vi "TCP Server - Parse message.vi"(6 "Sender IP":string, 8 "error in (no error)":errorcluster, 9 "Message":string, 10 "TCP Client ID":refnum<k5>, 11 "TCP Server in":refnum<class "TCP Server.lvclass">) -> (0 "error out":errorcluster, 1 "External error out":errorcluster, 3 "TCP Server out":refnum<class "TCP Server.lvclass">)   [LabVIEW 2026, in "TALOS.lvlib" / "TCP Server.lvlib" / "TCP Server.lvclass"]
uses:
  TCP Server.lvclass
  TCP Server Msg Actions.ctl
  Ancestor/Ancestor/Ancestor.lvclass/Ancestor.ctl
  <vilib>/Utility/error.llb/Trim Whitespace (string).vi
  <vilib>/Utility/error.llb/Trim Whitespace One-Sided.vi
  FGV/Error Memory/Get Error Description.vi
  Ancestor/Ancestor/Read ID.vi
  Support VIs/Get Class Name.vi
  <vilib>/Utility/error.llb/Clear Errors.vi
  FGV/Error Memory/Error Memory Core.vi
  <vilib>/AdvancedString/Delimited String to 1D String Array.vi
  <vilib>/AdvancedString/Delimited String to 1D String Array (string).vi
  Support VIs/Circus Root Path.vi
  FGV/Error Memory/Error Crt Lvl checker.vi
  FGV/Error Memory/Error Memory Core.vi/40c8088d-b597-4017-91af-faa98e00292e.vi
  FGV/Error Memory/Error Memory Core.vi/d4a3ab98-063c-4e44-b43d-fbdcfe6c2be2.vi
  Support VIs/Global Constants.vi
  Support VIs/Global Memory.vi
  <userlib>/_OpenG.lib/string/string.llb/Trim Whitespace (String)__ogtk.vi
  <vilib>/Utility/LVClass/Get LV Class Name.vi
  Support VIs/Is in Packed Library.vi
  Support VIs/TALOS Root path.vi
  Support VIs/Read CSV worksheet.vi
  <vilib>/Utility/error.llb/General Error Handler.vi
  Support VIs/Error Log.vi
  Ancestor/Ancestor/Ancestor.lvclass
  <vilib>/Comparison/Equal/Equal Functor/Equal Functor.lvclass
  bd90c6b7-bc86-460d-9dd7-41153e43b143.vi
  TALOS.lvlib
  <userlib>/_OpenG.lib/string/string.llb/openg_string.lvlib
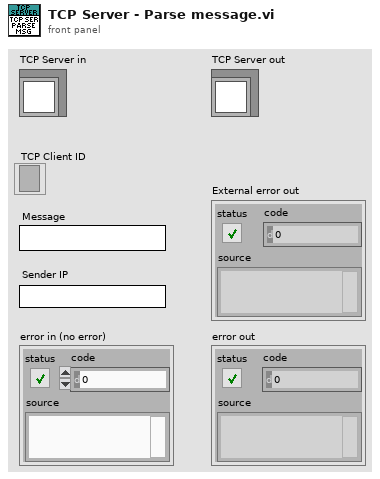
[diagram p1: front panel]
types:
  T1 = typedef "TALOS.lvlib/TCP Server.lvlib/TCP Server.lvclass/TCP Server Msg Actions.ctl" = enum16{"Spawn TCP Listener/Writer", "External Error", "I Exist", "Who the hell is this guy?", "Do nothing", "Are you the Bearer", "Farewell", "External Message"}
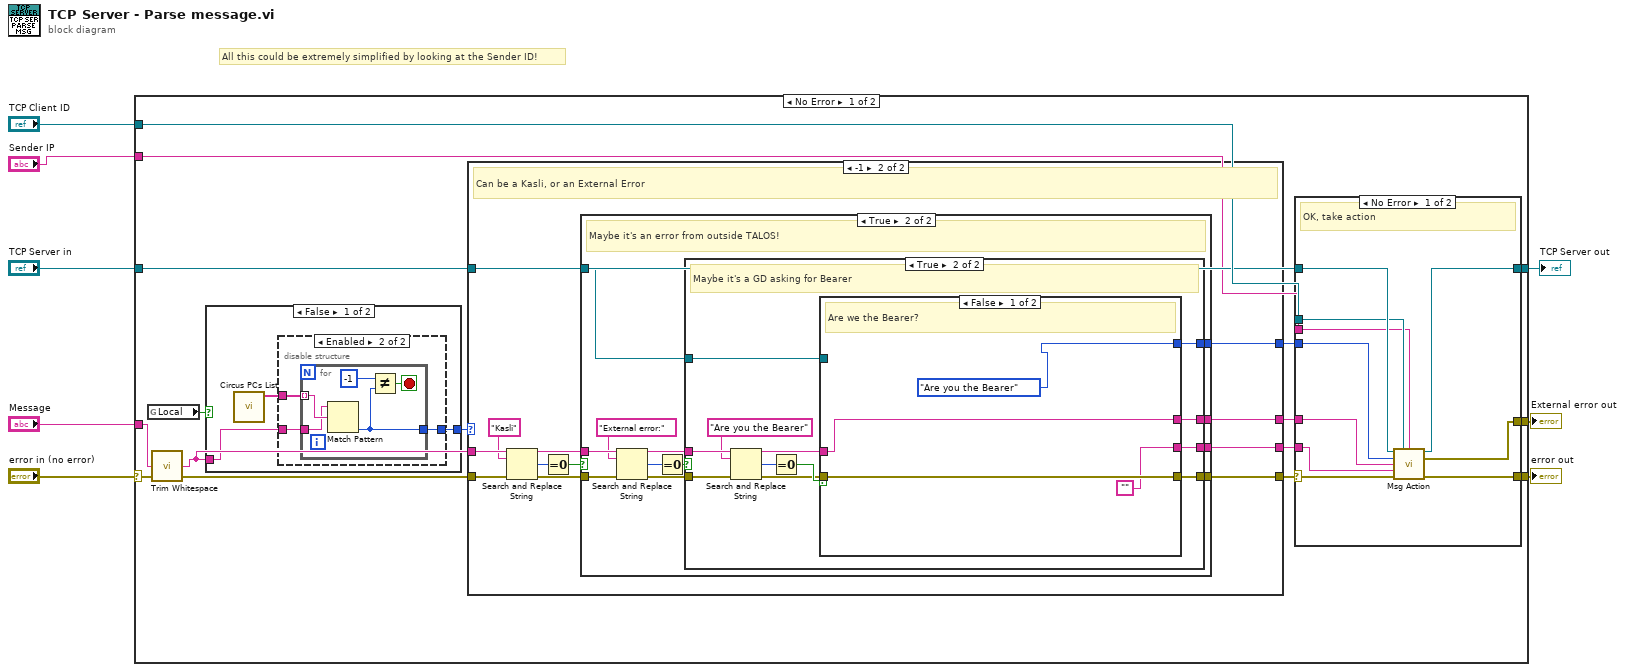
[diagram p0: block diagram]
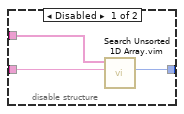
[diagram p2: hidden frame]
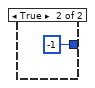
[diagram p3: hidden frame]
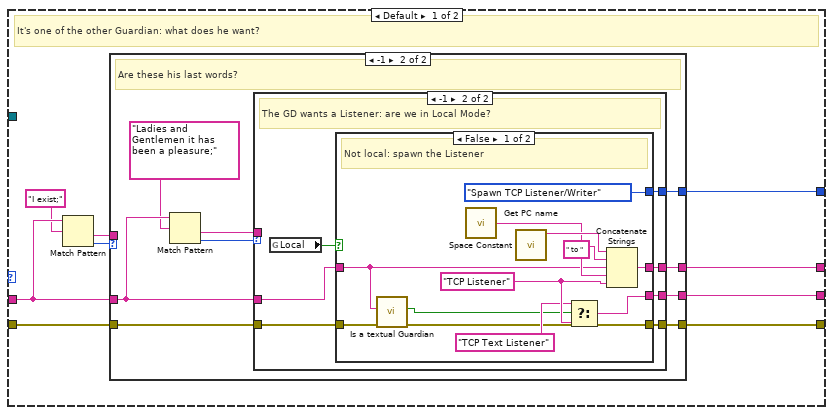
[diagram p4: hidden frame]
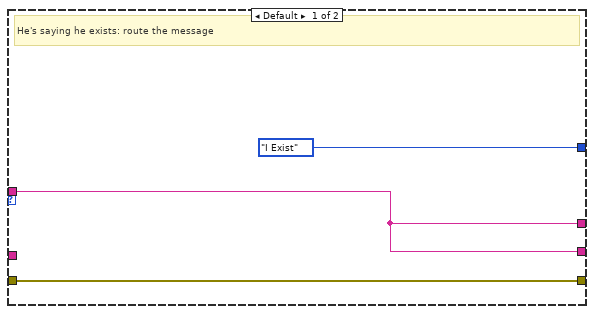
[diagram p5: hidden frame]
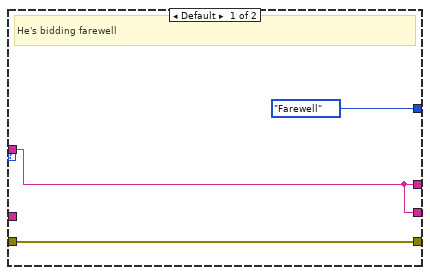
[diagram p6: hidden frame]
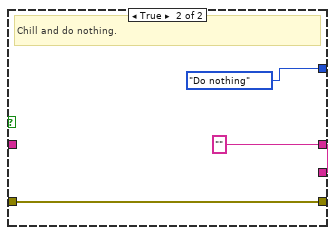
[diagram p7: hidden frame]
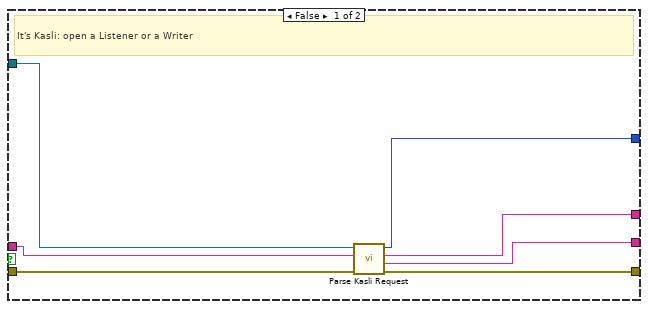
[diagram p8: hidden frame]
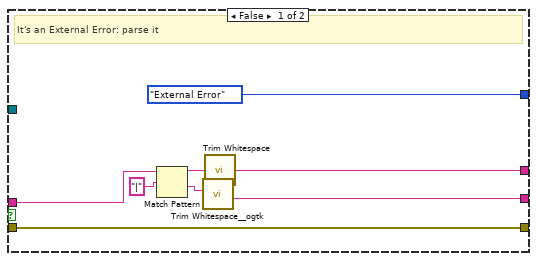
[diagram p9: hidden frame]
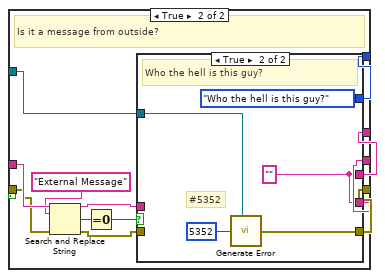
[diagram p10: hidden frame]
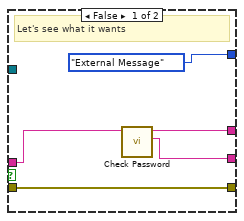
[diagram p11: hidden frame]
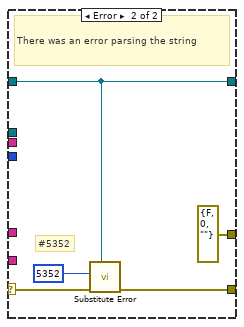
[diagram p12: hidden frame]
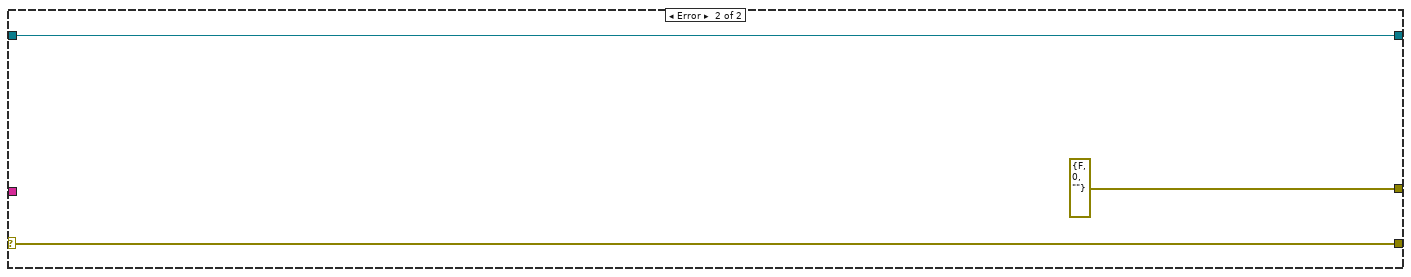
[diagram p13: hidden frame]
diagram:
  # "All this could be extremely simplified by looking at the Sender ID!"
  n1 = case shown="No Error" "error in (no error)" {
    selector: "error in (no error)" -> [w23 w178]
    tunnel: "Message" -> [w21 _]
    tunnel: "TCP Client ID" -> [w20 _]
    tunnel: [w19 w178] -> w5
    tunnel: "TCP Server in" -> [w18 w179]
    tunnel: [w14 w179] -> w3
    tunnel: [w12 errorcluster {"status"=FALSE, "code"=0, "source"=""} ("error out")] -> w2
    tunnel: "Sender IP" -> [w11 _]
    frame No Error {
      n2 = global read "Global Constants.vi" "Local"() -> (w9:bool)
      n3 = call-poly <vilib>:"Trim Whitespace.vi"("string"=w21) -> ("trimmed string"=w22:string)  [unwired: 1 in]
      n4 = case shown="False" w9 {
        tunnel: w22 -> [w26 _]
        tunnel: [w25 -1 ("offset past match")] -> w10
        frame False {
          n5 = call "Circus PCs List.vi"() -> ("PC List out"=w24:string[])  [unwired: 10 in, 1 out]
          n6 = disable-structure shown="Enabled" {
            disable-tunnel: w26 -> [w29 w32]
            disable-tunnel: [w28 w30] -> w25
            disable-tunnel: w24 -> [w27 w31]
            frame Disabled {
              n7 = call "Search Unsorted 1D Array.vim"("element"=w29, "unsorted 1D array"=w27) -> ("index of element"=w28:i32)  [unwired: 9 in]
            }
            frame Enabled {
              n8 = for {
                tunnel: w32 -> [w36]
                tunnel: w31 -> [w37] mode=indexing
                tunnel: [w34] -> w30
                stop <- w35 stop-if-true
                n9 = Match Pattern(string=w36, regular expression=w37) -> (offset past match=w34:i32)  [unwired: 1 in, 3 out]
                n10 = Not Equal?(x=-1, y=w34) -> (x != y?=w35:bool)
              }
            }
          }
        }
        frame True {
        }
      }
      n11 = case shown="-1" w10 {
        tunnel: [w47 w91] -> w17
        tunnel: w22 -> [w43 w95]
        tunnel: w23 -> [w46 w90]
        tunnel: [w45 w88] -> w16
        tunnel: w18 -> [_ w87]
        tunnel: [w44 w86] -> w15
        tunnel: [w41 w85] -> w13
        frame Default {
          # "It's one of the other Guardian: what does he want?"
          n12 = Match Pattern(string=w43, regular expression="I exist;") -> (after substring=w39:string, offset past match=w40:i32)  [unwired: 1 in, 2 out]
          n13 = case shown="-1" w40 {
            tunnel: [w50 w59] -> w47
            tunnel: w43 -> [_ w54]
            tunnel: w46 -> [w50 w58]
            tunnel: [w49 w57] -> w45
            tunnel: [w49 w56] -> w44
            tunnel: [TCP_Server_Msg_Actions."I Exist" w55] -> w41
            tunnel: w39 -> [w49 _]
            frame Default {
              # "He's saying he exists: route the message"
            }
            frame -1 {
              # "Are these his last words?"
              n14 = Match Pattern(string=w54, regular expression="Ladies and Gentlemen it has been a pleasure;" ("Message")) -> (after substring=w51:string, offset past match=w52:i32)  [unwired: 1 in, 2 out]
              n15 = case shown="-1" w52 {
                tunnel: [w61 w69] -> w59
                tunnel: w58 -> [w61 w68]
                tunnel: [w62 w67] -> w57
                tunnel: [w62 w65] -> w56
                tunnel: [TCP_Server_Msg_Actions."Farewell" w64] -> w55
                tunnel: w54 -> [_ w63]
                tunnel: w51 -> [w62 _]
                frame Default {
                  # "He's bidding farewell"
                }
                frame -1 {
                  # "The GD wants a Listener: are we in Local Mode?"
                  n16 = global read "Global Constants.vi" "Local"() -> (w66:bool)
                  n17 = case shown="False" w66 {
                    tunnel: [w73 w84] -> w69
                    tunnel: w63 -> [w72 _]
                    tunnel: w68 -> [w74 w84]
                    tunnel: [w78 w83] -> w67
                    tunnel: [w76 w83] -> w65
                    tunnel: [TCP_Server_Msg_Actions."Spawn TCP Listener/Writer" TCP_Server_Msg_Actions."Do nothing"] -> w64
                    frame False {
                      w77 = "TCP Listener" ("uService Class Name")
                      # "Not local: spawn the Listener"
                      n18 = call "Is a textual Guardian.vi"("error in (no error)"=w74, "Target GD ID"=w72) -> ("error out"=w73:errorcluster, "Textual?"=w71:bool)  [unwired: 8 in]
                      n19 = call <vilib>:"Space Constant.vi"() -> ("String"=w79:string)
                      n20 = call "Get PC name.vi"() -> ("Hostname"=w81:string)  [unwired: 10 in, 1 out]
                      n21 = Select(t="TCP Text Listener", s=w71, f=w77) -> (s? t:f=w76:string)
                      n22 = Concatenate Strings(w81, " to " ("string"), w72, w79, w77) -> (w78:string)
                    }
                    frame True {
                      w83 = ""
                      # "Chill and do nothing."
                    }
                  }
                }
              }
            }
          }
        }
        frame -1 {
          # "Can be a Kasli, or an External Error"
          n23 = Search and Replace String(input string=w95, search string="Kasli", error in=w90) -> (result string=w96:string, number of replacements=w93:i32, error out=w89:errorcluster)  [unwired: 5 in, 1 out]
          n24 = Equal To 0?(x=w93) -> (x = 0?=w92:bool)
          n25 = case shown="True" w92 {
            tunnel: [w102 w115] -> w91
            tunnel: w89 -> [w98 w110]
            tunnel: w96 -> [w99 w112]
            tunnel: [w100 w114] -> w88
            tunnel: w87 -> [w101 w104]
            tunnel: [w103 w109] -> w86
            tunnel: [w97 w105] -> w85
            frame False {
              # "It's Kasli: open a Listener or a Writer"
              n26 = call "Parse Kasli Request.vi"("error in (no error)"=w98, "Message part"=w99, "TCP Server in"=w101) -> ("error out"=w102:errorcluster, "uService Class Name"=w103:string, "uService ID"=w100:string, "TCP Server Msg Actions"=w97:T1)  [unwired: 5 in]
            }
            frame True {
              # "Maybe it's an error from outside TALOS!"
              n27 = Search and Replace String(input string=w112, search string="External error:", error in=w110) -> (result string=w107:string, number of replacements=w113:i32, error out=w106:errorcluster)  [unwired: 5 in, 1 out]
              n28 = Equal To 0?(x=w113) -> (x = 0?=w108:bool)
              n29 = case shown="True" w108 {
                tunnel: [w123 w135] -> w115
                tunnel: [w117 w134] -> w114
                tunnel: [w119 w125] -> w109
                tunnel: w107 -> [w121 w131]
                tunnel: w106 -> [w123 w130]
                tunnel: [TCP_Server_Msg_Actions."External Error" w133] -> w105
                tunnel: w104 -> [_ w124]
                frame False {
                  # "It's an External Error: parse it"
                  n30 = Match Pattern(string=w121, regular expression="|") -> (before substring=w118:string, after substring=w120:string)  [unwired: 1 in, 2 out]
                  n31 = call-poly <userlib>:"Trim Whitespace__ogtk.vi"("String in"=w120) -> ("String out"=w119:string)  [unwired: 6 in]
                  n32 = call-poly <vilib>:"Trim Whitespace.vi"("string"=w118) -> ("trimmed string"=w117:string)  [unwired: 1 in]
                }
                frame True {
                  # "Maybe it's a GD asking for Bearer"
                  n33 = Search and Replace String(input string=w131, search string="Are you the Bearer", error in=w130) -> (result string=w127:string, number of replacements=w132:i32, error out=w126:errorcluster)  [unwired: 5 in, 1 out]
                  n34 = Equal To 0?(x=w132) -> (x = 0?=w128:bool)
                  n35 = case shown="False" w128 {
                    tunnel: [w138 w151] -> w135
                    tunnel: [w139 w149] -> w134
                    tunnel: [TCP_Server_Msg_Actions."Are you the Bearer" w148] -> w133
                    tunnel: w127 -> [w139 w144]
                    tunnel: w126 -> [w138 w143]
                    tunnel: w124 -> [_ w150]
                    tunnel: ["" w140] -> w125
                    frame False {
                      # "Are we the Bearer?"
                    }
                    frame True {
                      # "Is it a message from outside?"
                      n36 = Search and Replace String(input string=w144, search string="External Message", error in=w143) -> (result string=w147:string, number of replacements=w146:i32, error out=w145:errorcluster)  [unwired: 5 in, 1 out]
                      n37 = Equal To 0?(x=w146) -> (x = 0?=w141:bool)
                      n38 = case shown="True" w141 {
                        tunnel: [w155 w160] -> w151
                        tunnel: w150 -> [_ w161]
                        tunnel: [w153 w158] -> w149
                        tunnel: [TCP_Server_Msg_Actions."External Message" TCP_Server_Msg_Actions."Who the hell is this guy?"] -> w148
                        tunnel: w147 -> [w156 _]
                        tunnel: w145 -> [w155 _]
                        tunnel: [w154 w158] -> w140
                        frame False {
                          # "Let's see what it wants"
                          n39 = call "Check Password.vi"("Message"=w156) -> ("Payload"=w154:string, "uService ID"=w153:string)  [unwired: 9 in]
                        }
                        frame True {
                          w158 = "" ("uService ID")
                          # "#5352"
                          # "Who the hell is this guy?"
                          n40 = call "Generate Error.vi"("Class"=w161, "Error Code"=5352) -> ("error out"=w160:errorcluster)  [unwired: 5 in]
                        }
                      }
                    }
                  }
                }
              }
            }
          }
        }
      }
      n41 = case shown="No Error" w17 {
        selector: w17 -> [w170 w176]
        tunnel: w20 -> [w166 _]
        tunnel: [w171 w175] -> w19
        tunnel: w18 -> [w167 w173]
        tunnel: w16 -> [w164 _]
        tunnel: w15 -> [w163 _]
        tunnel: [w169 w173] -> w14
        tunnel: w13 -> [w165 _]
        tunnel: [w168 errorcluster {"status"=FALSE, "code"=0, "source"=""} ("error out")] -> w12
        tunnel: w11 -> [w162 _]
        frame No Error {
          # "OK, take action"
          n42 = call "Msg Action.vi"("TCP Server in"=w167, "TCP Client ID"=w166, "Sender IP"=w162, "TCP Server Msg Actions"=w165, "uService ID"=w164, "uService Class Name"=w163, "error in (no error)"=w170) -> ("TCP Server out"=w169:refnum<class "TCP Server.lvclass">, "External Error out"=w168:errorcluster, "error out"=w171:errorcluster)  [unwired: 6 in]
        }
        frame Error {
          # "#5352"
          # "There was an error parsing the string"
          n43 = call "Substitute Error.vi"("LabVIEW Object"=w173, "error in (no error)"=w176, "Error Code"=5352) -> ("error out"=w175:errorcluster)  [unwired: 8 in]
        }
      }
    }
    frame Error {
    }
  }
  "error out" <- w5
  "TCP Server out" <- w3
  "External error out" <- w2
